vi "Initialize XNET Refs.vi"(8 "error in (no error)":errorcluster, 11 "XNET Settings":T1 {"FD ISO Mode" items=["ISO", "Non ISO", "ISO Legacy"]; "CAN I/O Mode" items=["CAN 2.0", "CAN FD", "CAN FD+BRS"]; "Termination" items=["Off", "On"]}) -> (0 "error out":errorcluster, 2 "Incoming":refnum<k21>, 3 "Outgoing":refnum<k21>)   [LabVIEW 2019, in "Ghost Bus Addon Engine.lvlib"]
uses:
  Ghost Bus Addon Engine.lvlib
  Addon Shared/Types/XNET Port Settings.ctl
  <vilib>/xnet/xnet.llb/XNET Create Session (Frame Output Stream).vi
  <vilib>/xnet/xnet.llb/XNET Create Session (Frame Input Stream).vi
  <resource>/objmgr/xnet.rc
  Addon Shared/Ghost Bus Addon Shared.lvlib
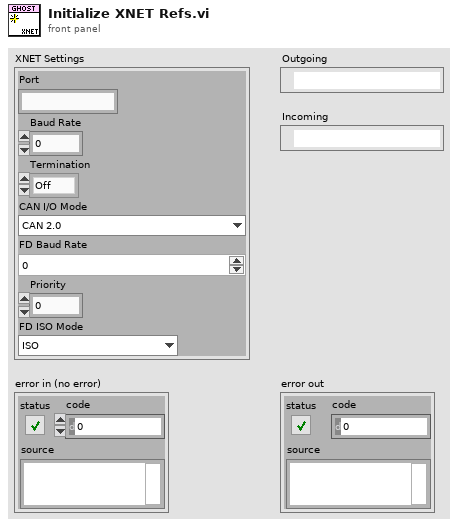
[diagram p1: front panel]
types:
  T1 = typedef "Ghost Bus Addon Shared.lvlib/XNET Port Settings.ctl" = cluster{"Port":string, "Baud Rate":u64, "Termination":u32, "CAN I/O Mode":u32, "FD Baud Rate":u64, "Priority":i32, "FD ISO Mode":u32}
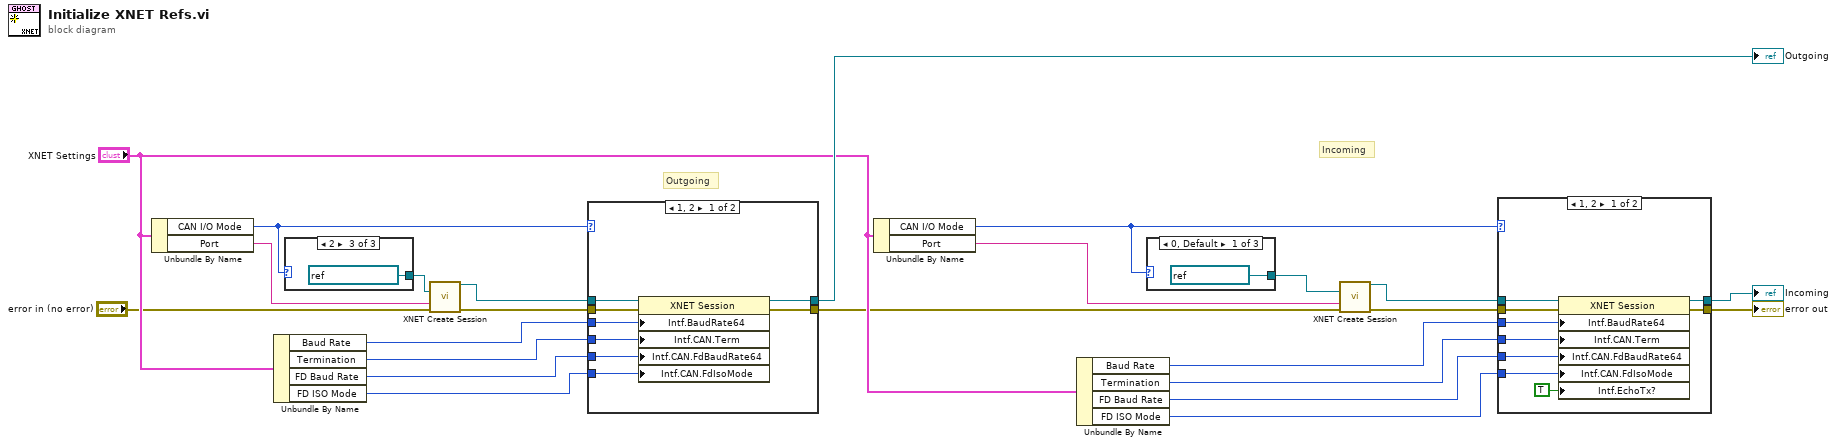
[diagram p0: block diagram]
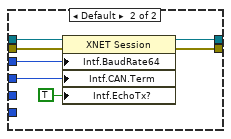
[diagram p2: hidden frame]
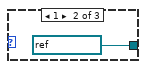
[diagram p3: hidden frame]
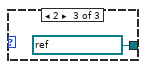
[diagram p4: hidden frame]
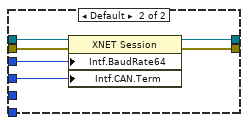
[diagram p5: hidden frame]
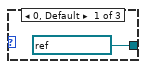
[diagram p6: hidden frame]
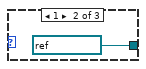
[diagram p7: hidden frame]
diagram:
  # "Incoming"
  # "Outgoing"
  n1 = Unbundle By Name("XNET Settings") -> ("CAN I/O Mode"=w7:u32, "Port"=w6:string)
  n2 = Unbundle By Name("XNET Settings") -> ("Baud Rate"=w9:u64, "Termination"=w10:u32, "FD Baud Rate"=w11:u64, "FD ISO Mode"=w12:u32)
  n3 = case shown="2" w7 {
    tunnel: [refnum<k21> ":memory:" ("cluster (:memory:)") refnum<k21> ":can_fd:" ("cluster (:memory:)") refnum<k21> ":can_fd_brs:" ("cluster (:memory:)")] -> w2
    frame 0, Default {
    }
    frame 1 {
    }
    frame 2 {
    }
  }
  n4 = call-poly <vilib>:"XNET Create Session.vi"("cluster (:memory:)"=w2, "interface"=w6, "error in (no error)"="error in (no error)") -> ("session out"=w3:refnum<k21>, "error out"=w1:errorcluster)  [unwired: 11 in]
  n5 = case shown="1, 2" w7 {
    tunnel: w1 -> [w35 w41]
    tunnel: w3 -> [w34 w40]
    tunnel: [w33 w39] -> w5
    tunnel: w11 -> [w32 _]
    tunnel: w10 -> [w31 w38]
    tunnel: w9 -> [w30 w37]
    tunnel: [w29 w36] -> w23
    tunnel: w12 -> [w28 _]
    frame 1, 2 {
      n6 = property class="XNET Session"(reference=w34, error in=w35, "Intf.BaudRate64"=w30, "Intf.CAN.Term"=w31, "Intf.CAN.FdBaudRate64"=w32, "Intf.CAN.FdIsoMode"=w28) -> (reference out=w29:refnum<k21>, error out=w33:errorcluster)
    }
    frame Default {
      n7 = property class="XNET Session"(reference=w40, error in=w41, "Intf.BaudRate64"=w37, "Intf.CAN.Term"=w38) -> (reference out=w36:refnum<k21>, error out=w39:errorcluster)
    }
  }
  "Outgoing" <- w23
  n8 = Unbundle By Name("XNET Settings") -> ("CAN I/O Mode"=w16:u32, "Port"=w17:string)
  n9 = Unbundle By Name("XNET Settings") -> ("Baud Rate"=w19:u64, "Termination"=w20:u32, "FD Baud Rate"=w21:u64, "FD ISO Mode"=w22:u32)
  n10 = case shown="0, Default" w16 {
    tunnel: [refnum<k21> ":memory:" ("cluster (:memory:)") refnum<k21> ":can_fd:" ("cluster (:memory:)") refnum<k21> ":can_fd_brs:" ("cluster (:memory:)")] -> w14
    frame 0, Default {
    }
    frame 1 {
    }
    frame 2 {
    }
  }
  n11 = call-poly <vilib>:"XNET Create Session.vi"("cluster (:memory:)"=w14, "interface"=w17, "error in (no error)"=w5) -> ("session out"=w13:refnum<k21>, "error out"=w15:errorcluster)  [unwired: 11 in]
  n12 = case shown="1, 2" w16 {
    tunnel: w15 -> [w53 w60]
    tunnel: w13 -> [w52 w59]
    tunnel: [w51 w58] -> w4
    tunnel: w21 -> [w50 _]
    tunnel: w20 -> [w49 w57]
    tunnel: w19 -> [w48 w56]
    tunnel: [w47 w55] -> w24
    tunnel: w22 -> [w46 _]
    frame 1, 2 {
      n13 = property class="XNET Session"(reference=w52, error in=w53, "Intf.BaudRate64"=w48, "Intf.CAN.Term"=w49, "Intf.CAN.FdBaudRate64"=w50, "Intf.CAN.FdIsoMode"=w46, "Intf.EchoTx?"=TRUE ("Interface:Echo Transmit?")) -> (reference out=w47:refnum<k21>, error out=w51:errorcluster)
    }
    frame Default {
      n14 = property class="XNET Session"(reference=w59, error in=w60, "Intf.BaudRate64"=w56, "Intf.CAN.Term"=w57, "Intf.EchoTx?"=TRUE ("Interface:Echo Transmit?")) -> (reference out=w55:refnum<k21>, error out=w58:errorcluster)
    }
  }
  "Incoming" <- w24
  "error out" <- w4
